vi "52-lfs-r4.vi"(8 "error in (no error)":errorcluster, 9 "Position in":T1) -> (0 "error out":errorcluster, 1 "Position out":T1)   [LabVIEW 2019]
uses:
  subVI/move/position cluster.ctl
  subVI/move control/move and align/move_cluster.ctl
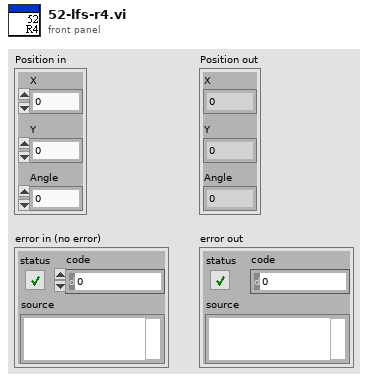
[diagram p1: front panel]
types:
  T1 = typedef "position cluster.ctl" = cluster{"X":dbl, "Y":dbl, "Angle":dbl}
  T2 = typedef "move_cluster.ctl" = cluster{"X":dbl, "Y":dbl, "degree":dbl, "speed":dbl}
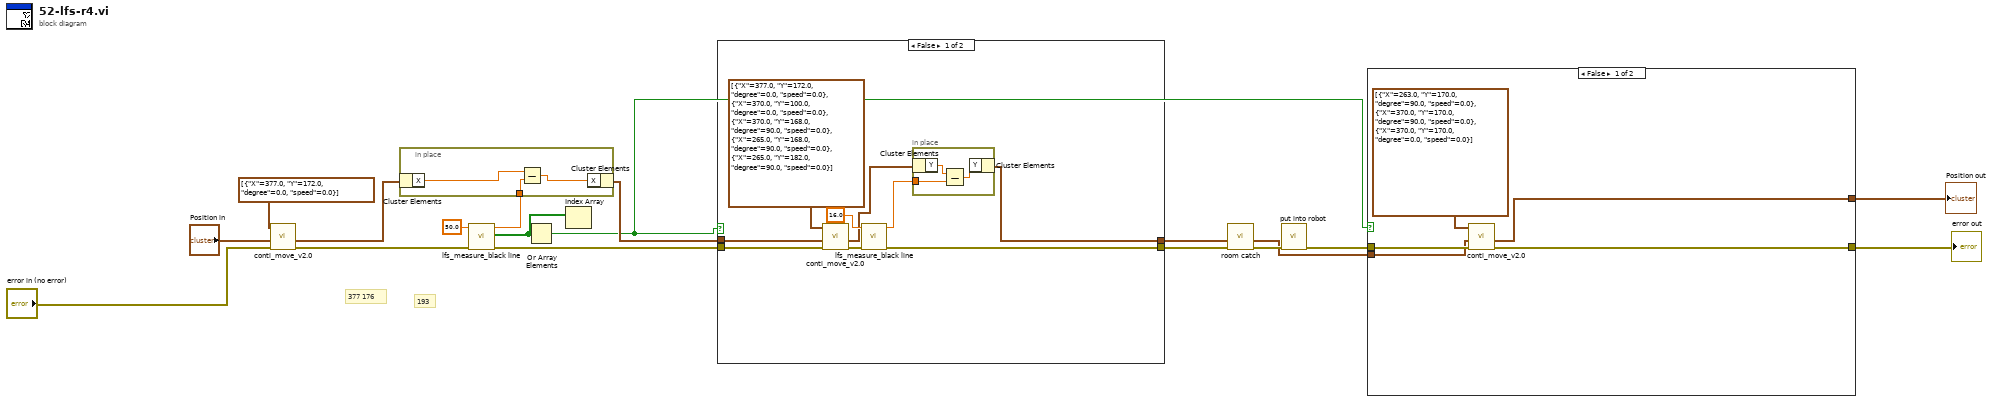
[diagram p0: block diagram]
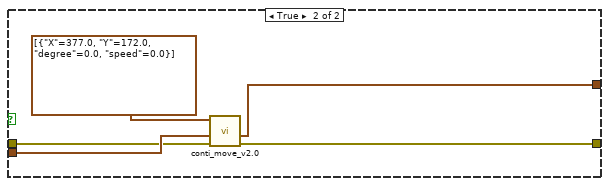
[diagram p2: hidden frame]
diagram:
  # "193"
  # "377 176"
  n1 = call "conti_move_v2.0.vi"("error in (no error)"="error in (no error)", "Position"="Position in", "route"=T2[] [{"X"=377.0, "Y"=172.0, "degree"=0.0, "speed"=0.0}]) -> ("error out"=w18:errorcluster, "Position out"=w13:T1)  [unwired: 7 in]
  n2 = call "lfs_measure_black line.vi"("error in (no error)"=w18, "limit"=50.0) -> ("error out"=w6:errorcluster, "0:R 1:L"=w11:bool[], "move cm"=w12:dbl)  [unwired: 7 in]
  n3 = in-place {
    in-place-border: w12 -> [w20]
    n4 = in-place-cluster #1(w13) -> ("X"=w21:dbl)
    n5 = Subtract(x=w21, y=w20) -> (x-y=w19:dbl)
    n6 = in-place-cluster #1("X"=w19) -> (w8:T1)
  }
  n7 = Or Array Elements(Boolean array=w11) -> (logical OR=w1:bool)
  n8 = Index Array(array=w11) -> ()  [unwired: 1 in, 1 out]
  n9 = case shown="False" w1 {
    tunnel: [w22 w35] -> w9
    tunnel: w8 -> [w28 w35]
    tunnel: [w23 w34] -> w7
    tunnel: w6 -> [w30 w34]
    frame False {
      n10 = call "conti_move_v2.0.vi"("error in (no error)"=w30, "Position"=w28, "route"=T2[] [{"X"=377.0, "Y"=172.0, "degree"=0.0, "speed"=0.0}, {"X"=370.0, "Y"=100.0, "degree"=0.0, "speed"=0.0}, {"X"=370.0, "Y"=168.0, "degree"=90.0, "speed"=0.0}, {"X"=265.0, "Y"=168.0, "degree"=90.0, "speed"=0.0}, {"X"=265.0, "Y"=182.0, "degree"=90.0, "speed"=0.0}]) -> ("error out"=w27:errorcluster, "Position out"=w25:T1)  [unwired: 7 in]
      n11 = call "lfs_measure_black line.vi"("error in (no error)"=w27, "limit"=16.0) -> ("error out"=w23:errorcluster, "move cm"=w24:dbl)  [unwired: 7 in, 1 out]
      n12 = in-place {
        in-place-border: w24 -> [w32]
        n13 = in-place-cluster #2(w25) -> ("Y"=w33:dbl)
        n14 = Subtract(x=w33, y=w32) -> (x-y=w31:dbl)
        n15 = in-place-cluster #2("Y"=w31) -> (w22:T1)
      }
    }
    frame True {
    }
  }
  n16 = call "room catch.vi"("error in (no error)"=w7, "Position in"=w9) -> ("error out"=w10:errorcluster, "Position out 2"=w5:T1)  [unwired: 8 in]
  n17 = call "put into robot.vi"("error in (no error)"=w10) -> ("error out"=w4:errorcluster)  [unwired: 10 in]
  n18 = case shown="False" w1 {
    tunnel: w5 -> [w39 w44]
    tunnel: w4 -> [w40 w43]
    tunnel: [w37 w42] -> w3
    tunnel: [w36 w41] -> w2
    frame False {
      n19 = call "conti_move_v2.0.vi"("error in (no error)"=w40, "Position"=w39, "route"=T2[] [{"X"=263.0, "Y"=170.0, "degree"=90.0, "speed"=0.0}, {"X"=370.0, "Y"=170.0, "degree"=90.0, "speed"=0.0}, {"X"=370.0, "Y"=170.0, "degree"=0.0, "speed"=0.0}]) -> ("error out"=w37:errorcluster, "Position out"=w36:T1)  [unwired: 7 in]
    }
    frame True {
      n20 = call "conti_move_v2.0.vi"("error in (no error)"=w43, "Position"=w44, "route"=T2[] [{"X"=377.0, "Y"=172.0, "degree"=0.0, "speed"=0.0}]) -> ("error out"=w42:errorcluster, "Position out"=w41:T1)  [unwired: 7 in]
    }
  }
  "Position out" <- w2
  "error out" <- w3
